vi "qmeter_io.vi"(11 "Sample type":u16) -> (1 "file path (dialog if empty) 3":path, 2 "file path (dialog if empty) 5":path, 3 "file path (dialog if empty) 4":path, 4 "file path (dialog if empty) 2":path, 5 "file path (dialog if empty)":path)   [LabVIEW 2019]
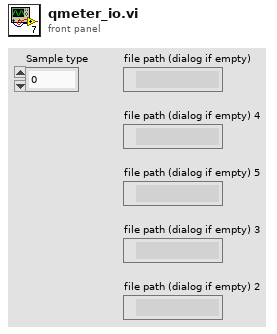
[diagram p1: front panel]
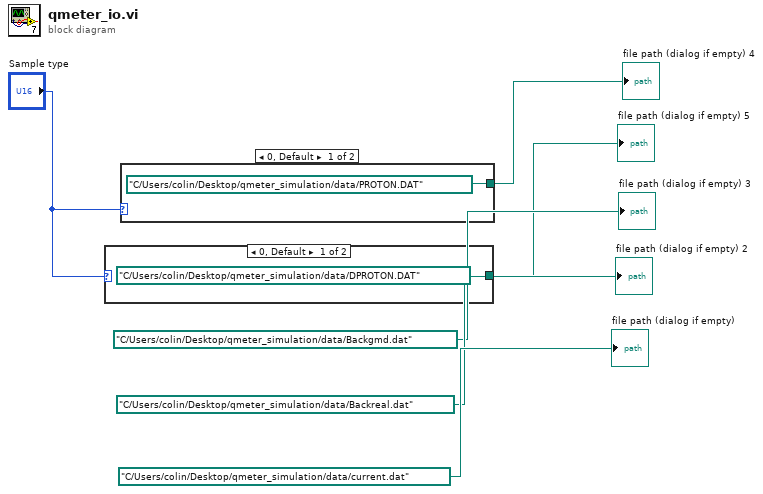
[diagram p0: block diagram]
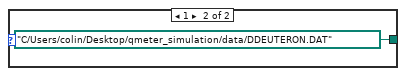
[diagram p2: hidden frame]
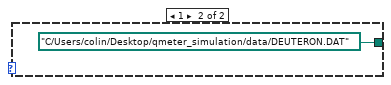
[diagram p3: hidden frame]
diagram:
  n1 = case shown="0, Default" "Sample type" {
    tunnel: [path "C:/Users/colin/Desktop/qmeter_simulation/data/DPROTON.DAT" ("file path (dialog if empty)") path "C:/Users/colin/Desktop/qmeter_simulation/data/DDEUTERON.DAT" ("file path (dialog if empty)")] -> w1
    frame 0, Default {
    }
    frame 1 {
    }
  }
  "file path (dialog if empty) 5" <- w1
  n2 = case shown="0, Default" "Sample type" {
    tunnel: [path "C:/Users/colin/Desktop/qmeter_simulation/data/PROTON.DAT" ("file path (dialog if empty)") path "C:/Users/colin/Desktop/qmeter_simulation/data/DEUTERON.DAT" ("file path (dialog if empty)")] -> w3
    frame 0, Default {
    }
    frame 1 {
    }
  }
  "file path (dialog if empty) 4" <- w3
  "file path (dialog if empty)" <- path "C:/Users/colin/Desktop/qmeter_simulation/data/current.dat" ("file path (dialog if empty)")
  "file path (dialog if empty) 2" <- path "C:/Users/colin/Desktop/qmeter_simulation/data/Backreal.dat" ("file path (dialog if empty)")
  "file path (dialog if empty) 3" <- path "C:/Users/colin/Desktop/qmeter_simulation/data/Backgmd.dat" ("file path (dialog if empty)")
